vi "HandleServers.vi"(8 "error in (no error)":errorcluster, 11 "S4ACS_GUI in":refnum<class "GuiderSetup.lvclass">) -> (0 "error out":errorcluster, 3 "S4ACS_GUI out":refnum<class "GuiderSetup.lvclass">)   [LabVIEW 2018, in "GuiderSetup.lvclass"]
uses:
  GuiderSetup.lvclass
  C:/Users/devstaff/sparc4/s4gui/Versao ZeroMQ REQ-REP/SPARC4_GUI -v1.0.0/S4GUI/S4GUI.lvclass
  S4GUI/S4GUI.lvclass/S4GUI.ctl
  Instrument/Instrument.lvclass
  S4GUI/S4GUI.lvclass
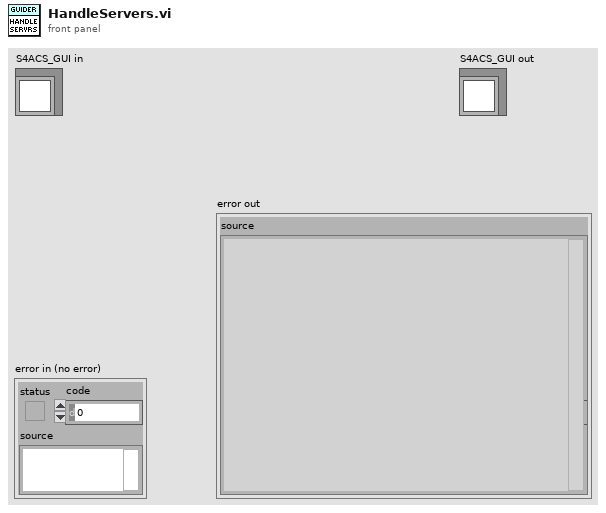
[diagram p1: front panel]
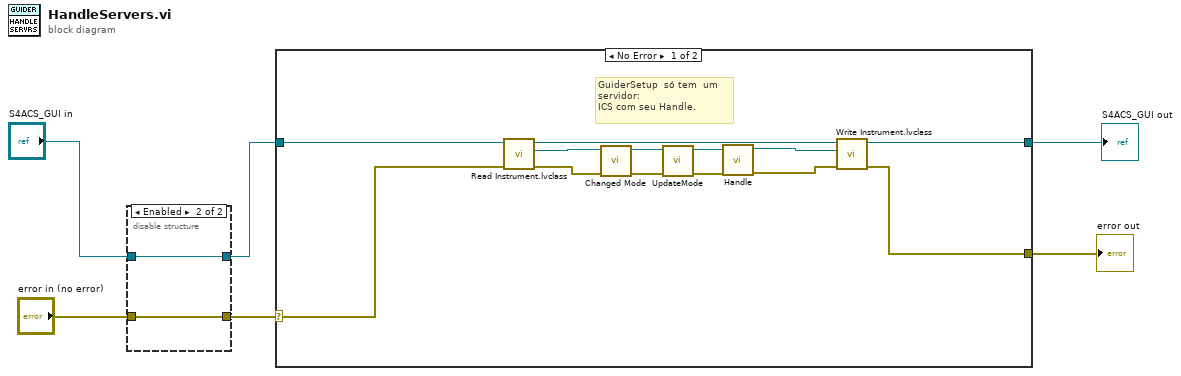
[diagram p0: block diagram]
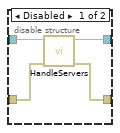
[diagram p3: hidden frame]
diagram:
  n1 = disable-structure shown="Enabled" {
    disable-tunnel: [w10 w11] -> w3
    disable-tunnel: [w9 w12] -> w4
    disable-tunnel: "error in (no error)" -> [w8 w11]
    disable-tunnel: "S4ACS_GUI in" -> [w7 w12]
    frame Disabled {
      n2 = call-parent "HandleServers.vi"("error in (no error)"=w8, "S4GUI in"=w7) -> ("error out"=w10:errorcluster, "S4GUI out"=w9:refnum<class "GuiderSetup.lvclass">)  [unwired: 8 in]
    }
    frame Enabled {
    }
  }
  n3 = case shown="No Error" w3 {
    selector: w3 -> [w22 w27]
    tunnel: [w13 w27] -> w1
    tunnel: [w14 w26] -> w2
    tunnel: w4 -> [w15 w26]
    frame No Error {
      # "GuiderSetup  só tem  um \nservidor:\nICS com seu Handle."
      n4 = call "Read Instrument.lvclass.vi"("error in (no error)"=w22, "S4ACS_GUI in"=w15) -> ("error out"=w18:errorcluster, "Instrument.lvclass"=w21:refnum<class "Instrument.lvclass">, "S4ACS_GUI out"=w23:refnum<class "GuiderSetup.lvclass">)  [unwired: 7 in]
      n5 = call-dynamic "Changed Mode.vi"("error in (no error)"=w18, "Instrument in"=w21) -> ("error out"=w17:errorcluster, "Instrument out"=w20:refnum<class "Instrument.lvclass">)  [unwired: 8 in]
      n6 = call-dynamic "UpdateMode.vi"("error in (no error)"=w17, "Instrument in"=w20) -> ("error out"=w16:errorcluster, "Instrument out"=w19:refnum<class "Instrument.lvclass">)  [unwired: 8 in]
      n7 = call-dynamic "Handle.vi"("error in (no error)"=w16, "Instrument in"=w19) -> ("error out"=w24:errorcluster, "Instrument out"=w25:refnum<class "Instrument.lvclass">)  [unwired: 8 in]
      n8 = call "Write Instrument.lvclass.vi"("error in (no error)"=w24, "Instrument.lvclass"=w25, "S4ACS_GUI in"=w23) -> ("error out"=w13:errorcluster, "S4ACS_GUI out"=w14:refnum<class "GuiderSetup.lvclass">)  [unwired: 7 in]
    }
    frame Error {
    }
  }
  "error out" <- w1
  "S4ACS_GUI out" <- w2
